vi "Read Condition.vi"(11 "IL U16 Allow in":refnum<class "IL U16 Pass.lvclass">) -> (2 "Allow":u16[](array[numeric]), 3 "IL U16 Allow out":refnum<class "IL U16 Pass.lvclass">)   [LabVIEW 2015, in "Interlocks.lvlib" / "IL U16 Pass.lvclass"]
uses:
  IL U16 Pass.lvclass
  IL U16 Pass.lvclass/IL U16 Pass.ctl
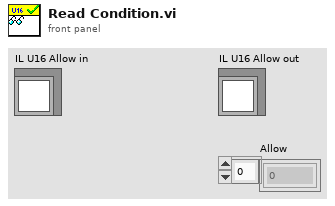
[diagram p1: front panel]
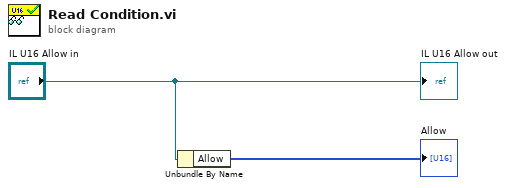
[diagram p0: block diagram]
diagram:
  n1 = Unbundle By Name("IL U16 Allow in") -> ("Allow"=→"Allow":u16[])
  "IL U16 Allow out" <- "IL U16 Allow in"
